vi "SpectrumSignalRecorder.vi"() -> (1 "error out":errorcluster, 3 "Intensity Signal":dbl[](array[numeric])=[2693.8, 2336.0, 2328.6, 2376.0, 2322.4, 2368.8, 2311.2, 2355.4, 2321.6, 2331.2, 2296.6, 2378.4, 2749.4, 2365.8, 2323.8, 2355.2, 2292.4, 2359.4, 2307.6, 2320.0, 2301.4, 2363.4, 2351.6, 2320.8, 2357.2, 2346.8, 2324.8, 2578.8, 2311.4, 2371.8, 2313.8, 2406.8, 2378.0, 2329.4, 2606.4, 2329.0, 2276.6, 2362.4, 3364.6, 2344.2, 2343.8, 2397.6, 2319.2, 2389.4, 2321.0, 2391.2, 2282.6, 2503.4, 2370.6, 2450.0, 2312.0, 2414.2, 2333.8, 2662.2, 2363.6, 2426.8, 2356.8, 2392.6, 2360.4, 2352.2, 2551.4, 2399.2, 2335.2, 2396.6, 2350.2, 2407.4, 2340.2, 2402.2, 2493.2, 2441.0, 2356.6, 2495.4, 2436.8, 2370.4, 2346.8, 2395.2, 2354.0, 2418.0, 2310.2, 2386.4, 2323.0, 2379.6, 2431.2, 2366.0, 2334.2, 2365.4, 2317.6, 2395.4, 2319.4, 2345.2, 2342.8, 2391.6, 2894.2, 2475.6, 2309.4, 2388.0, 2320.4, 2389.0, 2303.0, 2362.4, 2339.6, 2363.4, 2354.8, 2461.6, 2399.4, 2376.2, 2347.8, 2337.2, 3350.4, 2378.6, 2289.4, 2442.4, 2308.6, 2389.4, 2332.2, 2398.0, 2359.4, 2382.0, 2299.4, 2488.6, 2294.4, 2312.6, 2290.0, 2368.6, 2304.2, 2398.6, 2329.2, 2423.8, 2414.4, 2375.2, 2363.4, 2363.8, 2327.4, 2514.4, 2315.4, 2368.0, 2314.4, 2358.8, 2359.2, 2343.4, 2329.8, 2381.2, 2269.8, 2583.8, 2315.0, 2791.0, 2351.0, 2367.4, 2309.2, 2337.4, 2334.0, 2306.0, 2313.2, 2339.2, 2296.2, 2371.0, 2306.8, 2343.2, 2336.8, 2434.4, 2313.6, 2400.0, 2334.8, 2353.4, 2319.8, 2332.4, 2356.6, 2374.0, 2333.4, 2399.0, 2323.8, 2331.0, 2432.6, 2353.6, 2329.6, 2335.0, 2330.6, 2342.0, 2333.4, 2346.6, 2327.6, 2342.8, 2302.6, 2371.2, 2354.4, 2362.2, 2295.4, 2321.2, 2322.0, 2341.8, 2386.4, 2369.2, 2302.2, 2356.4, 2340.6, 2358.0, 2325.8, 2355.6, 2287.0, 2387.8, 2337.8, 2317.4, 2352.0, 2371.0, 2331.6, 2371.2, 2329.4, 2468.6, 2271.0, 2404.2, 2317.2, 2545.0, 2497.2, 2403.8, 2333.2, 2366.6, 2335.2, 2382.8, 2332.0, 3347.4, 2359.2, 2410.6, 2324.6, 2350.6, 2332.2, 2323.6, 2320.4, 2362.0, 2309.4, 2371.6, 2330.2, 2371.8, 2338.2, 2341.8, 2339.6, 2371.6, 2330.8, 2375.6, 2314.2, 2359.8, 2309.6, 2442.6, 2305.0, 2372.8, 2291.4, 2378.4, 2379.4, 2330.6, 2356.6, 2361.8, 2363.0, 2410.0, 2342.2, 2358.8, 2311.4, 2388.8, 2321.2, 2627.4, 2427.0, 2558.0, 2359.0, 2406.4, 2302.4, 2352.4, 2293.4, 2377.4, 3271.2, 2380.0, 2358.2, 2398.0, 3385.6, 2747.8, 2350.2, 2365.6, 2356.8, 2411.2, 2372.0, 2407.8, 2680.4, 2341.8, 2365.4, 2406.6, 2329.6, 2492.4, 2325.2, 2404.4, 3861.4, 2411.0, 2368.6, 2365.8, 2335.4, 2409.4, 2362.4, 2383.4, 2327.2, 2398.4, 2358.6, 2410.0, 2547.4, 2418.0, 2489.0, 2652.6, 2637.8, 2790.4, 2858.4, 2837.4, 2763.2, 2868.0, 2594.8, 2554.4, 2432.0, 2478.8, 2375.8, 2463.0, 2365.8, 2421.8, 2342.0, 2406.4, 2378.6, 2396.6, 2377.4, 2400.2, 2384.0, 2389.8, 2361.4, 2387.4, 2363.0, 2375.6, 2512.2, 2439.6, 2399.0, 2417.2, 2412.8, 3104.4, 2383.6, 2389.2, 2364.6, 2410.0, 2371.4, 2421.8, 2382.0, 2392.8, 2735.0, 2441.6, 2404.6, 2418.0, 2365.2, 2448.2, 2355.4, 2502.4, 2390.4, 2892.4, 2384.0, 2426.6, 2388.4, 2406.0, 2495.2, 2469.4, 2391.8, 2431.0, 2369.2, 2446.4, 2425.8, 2454.8, 2409.4, 2492.0, 2400.4, 2718.6, 3402.0, 3660.4, 3911.8, 4326.0, 4450.4, 4421.0, 4076.4, 3834.0, 3509.4, 3324.6, 3039.0, 2872.8, 2704.2, 2688.0, 2619.6, 2608.4, 2571.4, 2594.6, 2543.4, 2610.8, 2614.4, 2675.2, 2599.8, 2688.8, 2638.0, 2684.6, 2637.6, 2670.4, 2654.4, 2707.6, 2674.0, 2695.2, 2695.8, 2754.2, 2667.6, 2800.0, 3033.0, 2775.2, 2733.8, 2835.4, 2777.2, 2868.6, 2843.8, 2823.8, 2738.4, 2937.0, 2800.6, 2845.0, 2889.0, 2871.0, 2844.8, 3053.6, 3573.6, 4761.0, 5459.6, 6227.4, 6755.6, 7178.8, 6789.2, 6009.4, 5412.0, 4681.0, 4159.4, 3644.4, 3303.2, 3130.8, 2987.0, 3110.2, 3008.4, 3008.6, 2954.8, 2952.4, 5080.8, 2954.2, 3027.4, 2943.2, 3098.4, 2980.2, 2966.6, 2968.0, 2932.4, 3051.6, 3039.2, 2915.0, 2944.4, 3093.2, 2933.6, 3054.4, 2933.0, 3238.4, 2917.0, 2964.8, 2868.4, 2924.8, 2938.8, 3683.2, 2944.4, 2907.4, 2980.6, 2909.2, 2866.2, 2886.8, 3059.0, 2861.0, 3172.6, 2907.2, 2847.4, 2901.8, 2886.2, 2881.6, 2857.0, 3337.6, 2824.2, 2827.8, 2806.6, 2919.0, 2804.8, 2829.6, 2848.8, 2840.0, 2907.8, 2848.0, 2747.4, 2814.0, 3193.4, 2841.6, 2766.4, 2858.8, 2724.6, 2827.6, 2778.6, 2841.2, 2868.0, 3231.0, 3021.2, 3192.6, 3213.4, 3422.8, 3497.4, 4283.2, 3797.8, 3950.4, 3900.0, 3989.8, 3941.8, 5328.0, 3948.4, 3969.0, 3914.0, 4019.8, 3806.8, 3835.0, 3753.4, 3744.4, 3637.6, 3625.2, 3467.0, 3398.8, 3379.2, 3373.2, 3295.6, 3312.6, 3256.8, 3164.8, 3111.6, 3103.0, 2974.6, 2956.4, 2846.0, 2885.2, 2796.2, 2846.6, 3046.4, 2720.6, 2685.8, 2673.0, 2958.2, 2736.8, 2621.6, 2694.0, 2644.2, 2696.8, 2602.2, 2694.0, 2696.6, 2666.0, 2693.4, 3324.0, 2611.2, 2647.0, 2616.8, 2883.6, 2595.4, 2633.6, 2616.4, 2670.6, 2611.4, 2657.0, 2606.2, 2663.8, 2613.0, 2710.4, 2593.8, 2678.8, 2716.2, 2626.4, 2689.4, 2615.4, 2586.2, 2777.6, 2627.2, 2635.4, 2633.4, 2681.4, 2780.6, 2697.0, 2716.0, 2746.6, 2739.0, 2834.4, 2811.6, 2936.8, 3058.2, 3186.6, 3346.6, 3553.6, 3786.8, 4183.8, 4567.0, 5189.6, 5768.0, 6290.0, 6709.8, 7168.8, 7250.6, 7665.6, 8287.4, 9381.8, 9427.6, 9854.4, 10037.2, 9757.6, 9216.6, 8524.8, 7756.4, 7128.0, 6404.4, 5781.2, 5296.0, 4762.4, 4259.4, 4062.0, 3707.4, 3613.6, 3394.4, 3265.0, 3125.0, 3051.4, 3013.2, 2875.6, 2790.6, 2763.4, 2812.4, 2764.8, 2672.4, 2792.4, 2656.0, 2695.2, 2637.2, 2701.6, 2903.6, 2640.4, 2851.4, 2706.8, 2666.6, 2662.4, 2594.4, 2683.6, 2735.8, 2648.0, 2640.0, 2645.6, 2583.0, 2602.6, 2559.0, 2690.6, 2702.4, 2830.0, 2906.0, 3028.4, 3132.2, 3331.6, 3551.2, 3467.2, 3409.8, 3518.4, 3424.8, 3495.2, 3458.2, 3485.4, 3426.8, 3513.2, 3456.4, 3675.6, 3616.0, 3865.0, 3704.6, 3731.0, 3722.6, 3689.0, 3575.4, 3589.4, 3549.4, 3526.6, 3490.4, 3459.8, 3394.2, 3371.6, 3233.0, 3334.0, 3155.2, 3089.4, 3028.4, 3029.6, 3006.4, 3452.8, 2979.6, 2984.4, 2890.4, 2912.4, 2847.8, 2836.0, 2802.4, 2818.2, 2905.6, 2810.0, 2893.4, 2854.2, 2818.4, 2985.2, 3103.8, 3579.8, 4181.8, 4824.2, 5529.4, 6156.8, 6423.2, 6433.2, 6220.2, 6022.0, 5734.4, 5425.4, 4925.2, 4508.2, 4190.2, 3978.0, 3733.4, 4218.4, 3353.6, 3275.2, 3200.0, 3176.8, 3154.8, 3163.0, 3110.8, 3111.4, 3102.6, 3209.2, 3079.6, 3121.2, 3109.4, 3101.0, 3058.2, 3176.0, 4345.2, 3177.4, 3312.2, 3187.6, 3195.8, 3100.4, 2991.0, 2969.6, 2908.0, 2868.0, 2783.8, 2783.2, 2747.0, 2689.8, 2612.0, 2651.0, 2623.8, 2734.6, 2630.2, 2705.0, 2656.0, 2652.4, 2593.8, 2647.6, 2623.4, 2627.4, 2605.8, 2634.8, 2583.6, 2643.2, 2604.2, 2637.2, 2594.8, 2672.2, 2634.0, 2689.2, 2634.6, 2678.2, 2648.2, 2679.4, 2603.2, 2624.4, 2602.6, 2750.8, 2626.8, 2598.0, 2607.2, 2619.2, 2595.0, 2780.0, 2547.0, 2622.2, 3205.8, 2660.6, 2616.8, 2615.0, 2599.6, 2637.4, 2596.8, 2594.2, 2573.0, 2568.4, 2530.4, 2605.4, 2553.8, 2585.2, 2555.8, 2633.4, 2530.6, 2574.0, 2494.4, 2583.0, 2565.4, 2626.0, 2567.0, 2620.2, 2542.4, 2594.8, 2545.2, 2568.8, 2526.2, 2586.6, 2559.0, 2587.4, 2559.4, 2561.8, 2605.6, 2558.8, 2540.2, 2556.6, 2595.6, 2569.6, 2832.8, 2642.0, 2573.8, 2576.4, 2565.4, 2717.0, 2645.2, 2602.0, 2569.6, 2651.6, 2587.4, 2584.8, 3887.0, 2590.6, 2584.2, 2606.0, 2497.8, 2542.2, 2518.6, 2552.2, 2495.0, 2550.8, 2534.2, 2570.2, 2533.6, 2529.2, 2558.6, 2580.6, 2922.6, 2639.0, 2654.0, 2668.4, 2645.6, 2776.8, 2741.4, 2789.6, 2741.4, 2744.4, 2757.8, 2764.8, 2716.0, 2772.2, 2707.4, 2945.2, 2760.0, 2617.8, 2577.6, 2560.2, 2531.8, 2532.2, 2535.0, 2497.0, 2665.8, 2581.8, 2522.6, 2514.6, 2498.0, 2508.4, 2513.0, 2518.4, 2503.6, 2518.8, 2515.6, 2596.0, 2509.2, 2506.4, 2495.2, 2543.8, 2473.6, 2589.4, 2523.4, 2539.6, 2511.8, 2533.0, 2459.8, 3530.0, 2488.0, 2541.4, 2678.0, 2653.2, 2523.8, 2522.8, 2528.8, 2549.0, 2537.8, 2560.0, 2497.2, 2522.4, 2497.8, 2555.6, 2509.0, 2549.8, 2507.6, 2665.4, 2526.4, 2528.6, 2554.4, 2561.4, 2561.2, 2583.4, 2529.0, 2538.0, 2498.2, 2551.0, 2477.8, 2523.2, 2542.4, 2541.8, 2525.8, 2524.2, 2493.8, 2550.4, 2511.2, 2546.4, 2479.8, 2571.8, 2484.4, 2498.0, 2479.6, 2514.2, 2519.6, 2447.2, 2485.0, 2474.0, 2462.2, 2499.0, 2479.0, 2490.0, 2481.8, 2504.6, 2455.6, 2526.4, 2504.6, 2504.0, 2495.2, 2522.4, 2488.6, 2529.6, 2503.8, 2548.8, 2504.6, 2599.6, 2554.0, 2561.0, 2500.4, 2561.4, 2523.6, 2788.6, 2484.6, 2515.4, 2466.2, 2526.4, 2534.8, 2535.6, 2514.8, 2546.0, 2464.6, 2708.4, 2506.2, 2522.2, 2634.0, 2535.4, 2467.2, 2540.0, 2446.8, 2593.2, 2465.4, 2513.6, 2462.0, 2527.0, 2483.6, 2520.0, 2447.6, 2513.6, 2477.6, 2515.2, 3050.0, 2503.4, 2539.0, 2526.4, 2489.8, 2502.6, 2455.4, 2507.8, 2476.2, 2563.4, 2643.6, 2519.4, 2412.0, 2717.8])   [LabVIEW 2019]
uses:
  Dependencies/Controls/specu1a 1.0.0 Parameters.ctl
  Dependencies/Controls/specu1a 1.0.0 Trigger Edge.ctl
  Dependencies/Controls/specu1a 1.0.0 Trigger Mode.ctl
panel:
  in  "milliseconds to wait":u32=2000
  out "OKPH":bool=TRUE
  out "PipeHandle":i32
  in  "Parameters":T1={"Integration time"=1000000, "Gain"=enum."High", "TriggerEdge"=enum."Rising", "Trigger Mode"=enum."Internal", "Reserved"=0}
  out "DeviceHandle":i32
  out "OKDH":bool=TRUE
  in  "average":i32=6
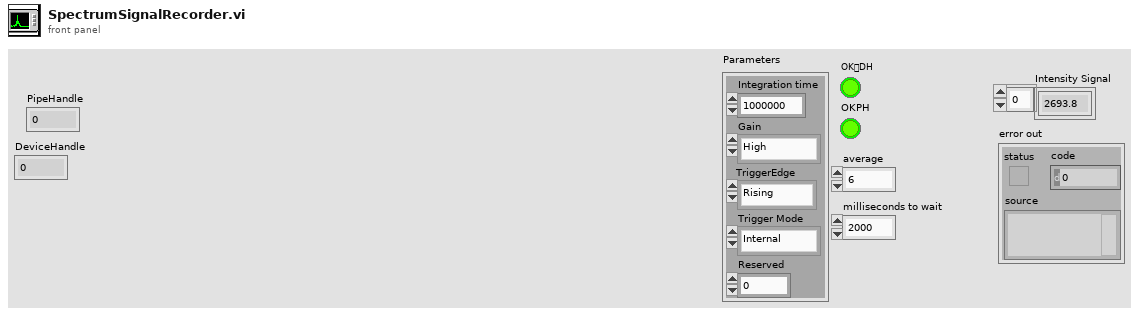
[diagram p1: front panel]
types:
  T1 = typedef "specu1a 1.0.0 Parameters.ctl" = cluster{"Integration time":u32, "Gain":enum16{"Low", "High", "No Function"}, "TriggerEdge":T2, "Trigger Mode":T3, "Reserved":u8}
  T2 = typedef "specu1a 1.0.0 Trigger Edge.ctl" = enum16{"Rising", "Falling", "No Function"}
  T3 = typedef "specu1a 1.0.0 Trigger Mode.ctl" = enum16{"Internal", "Asynchronous", "Synchronous"}
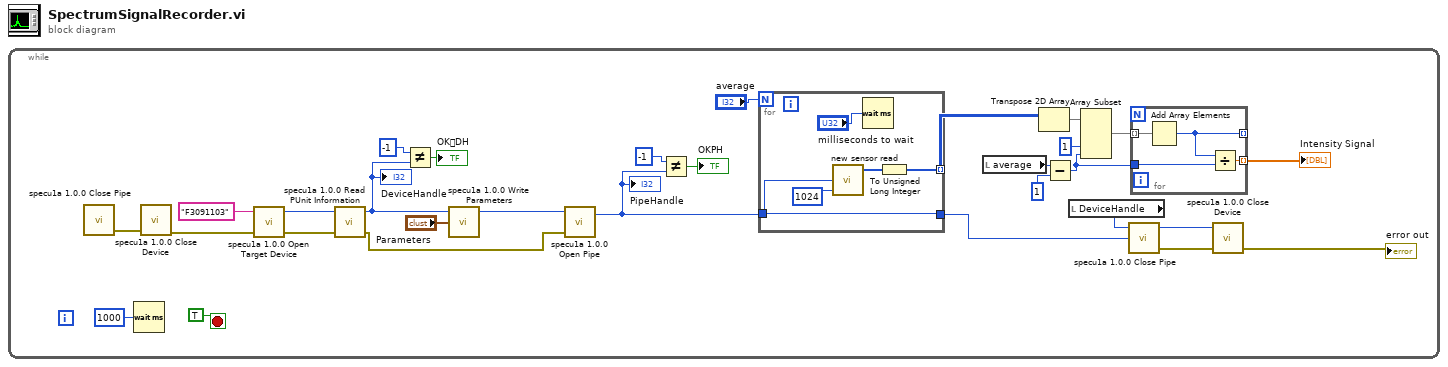
[diagram p0: block diagram]
diagram:
  n1 = while {
    stop <- TRUE ("stop") stop-if-true
    n2 = call "specu1a 1.0.0 Close Pipe.vi"() -> ("error out"=w8:errorcluster)  [unwired: 4 in, 1 out]
    n3 = Wait (ms)(milliseconds to wait=u32 1000) -> ()  [unwired: 1 out]
    n4 = call "specu1a 1.0.0 Close Device.vi"("error in (no error)"=w8) -> ("error out"=w7:errorcluster)  [unwired: 4 in]
    n5 = call "specu1a 1.0.0 Open Target Device.vi"("error in"=w7, "Unit ID"="F3091103") -> ("error out"=w25:errorcluster, "Device Handle"=w26:i32)  [unwired: 1 in, 1 out]
    n6 = call "specu1a 1.0.0 Read PUnit Information.vi"("error in (no error)"=w25, "Device Handle"=w26) -> ("error out"=w9:errorcluster, "Device Handle out"=w20:i32)  [unwired: 1 in, 1 out]
    "DeviceHandle" <- w20
    n7 = Not Equal?(x=-1, y=w20) -> (x != y?=→"OKDH":bool)
    n8 = call "specu1a 1.0.0 Write Parameters.vi"("Parameters"="Parameters", "Device Handle"=w20) -> ("Device Handle out"=w10:i32)  [unwired: 2 in, 1 out]
    n9 = call "specu1a 1.0.0 Open Pipe.vi"("error in (no error)"=w9, "Device Handle"=w10) -> ("Pipe Handle"=w19:i32)  [unwired: 1 in, 2 out]
    "PipeHandle" <- w19
    n10 = Not Equal?(x=-1, y=w19) -> (x != y?=→"OKPH":bool)
    n11 = for {
      N: "average" -> [_]
      tunnel: [w35] -> w18 mode=indexing
      tunnel: w19 -> [w31]
      tunnel: [w31] -> w2
      n12 = call "new sensor read.vi"("Pipe handle"=w31, "PixelSize"=u16 1024) -> ("Data buffer"=w32:u16[])  [unwired: 4 in, 3 out]
      n13 = Wait (ms)(milliseconds to wait="milliseconds to wait") -> ()  [unwired: 1 out]
      n14 = To Unsigned Long Integer(number=w32) -> (unsigned 32bit integer=w35:u32[])
    }
    n15 = local read "average"() -> (w3:i32)
    n16 = Transpose 2D Array(2D array=w18) -> (transposed array=w17:u32[][])
    n17 = Subtract(x=w3, y=1) -> (x-y=w12:i32)
    n18 = local read "DeviceHandle"() -> (w5:i32)
    n19 = Array Subset(array=w17, index (col)=1 ("index"), length (col)=w12) -> (w13:u32[][])  [unwired: 2 in]
    n20 = call "specu1a 1.0.0 Close Pipe.vi"("Pipe Handle"=w2, "Device Handle"=w5) -> ("error out"=w4:errorcluster, "Device Handle out"=w6:i32)  [unwired: 2 in]
    n21 = for {
      tunnel: w13 -> [w39] mode=indexing
      tunnel: [w38] -> _ mode=indexing
      tunnel: [w37] -> w11 mode=indexing
      tunnel: w12 -> [w36]
      n22 = Add Array Elements(numeric array=w39) -> (sum=w38:u32)
      n23 = Divide(x=w38, y=w36) -> (x/y=w37:dbl)
    }
    "Intensity Signal" <- w11
    n24 = call "specu1a 1.0.0 Close Device.vi"("error in (no error)"=w4, "Device Handle"=w6) -> ("error out"=→"error out":errorcluster)  [unwired: 3 in]
  }
